vi "night time stamp.vi"(8 "error in (no error)":errorcluster) -> (0 "error out":errorcluster, 2 "date time rec":T1)   [LabVIEW 2018]
uses:
  <vilib>/Utility/miscctls.llb/LVDateTimeRec.ctl
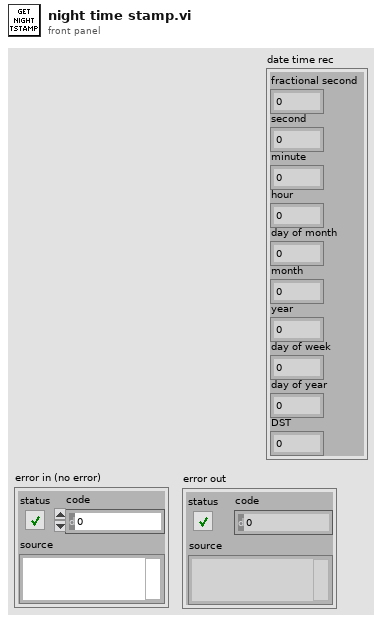
[diagram p1: front panel]
types:
  T1 = typedef "LVDateTimeRec.ctl" = cluster{"fractional second":dbl, "second":i32, "minute":i32, "hour":i32, "day of month":i32, "month":i32, "year":i32, "day of week":i32, "day of year":i32, "DST":i32}
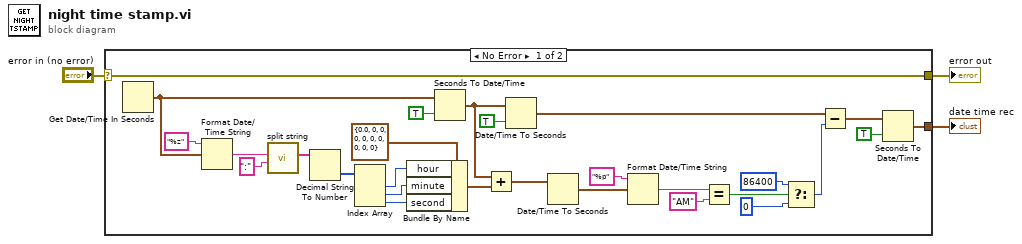
[diagram p0: block diagram]
diagram:
  n1 = case shown="No Error" "error in (no error)" {
    selector: "error in (no error)" -> [w31 w32]
    tunnel: [w31 w32] -> w2
    tunnel: [w6 _] -> w1
    frame No Error {
      n2 = Get Date/Time In Seconds() -> (seconds since 1Jan1904=w21:timestamp)
      n3 = Format Date/Time String(time format string (%c)="%z", seconds (now)=w21) -> (date/time string=w28:string)  [unwired: 1 in]
      n4 = call "split string.vi"("search string"=":", "String"=w28) -> ("strings array"=w26:string[])  [unwired: 8 in, 1 out]
      n5 = Decimal String To Number(string=w26) -> (number=w25:i32[])  [unwired: 2 in, 1 out]
      n6 = Index Array(array=w25) -> (element #1=w24:i32, element #2=w23:i32, element #3=w22:i32)  [unwired: 3 in]
      n7 = Bundle By Name(cluster=T1 {"fractional second"=0.0, "second"=0, "minute"=0, "hour"=0, "day of month"=0, "month"=0, "year"=0, "day of week"=0, "day of year"=0, "DST"=0} ("date time rec 2"), "hour"=w24, "minute"=w23, "second"=w22) -> (w19:T1)
      n8 = Seconds To Date/Time(time stamp (now)=w21, to UTC (F)=TRUE) -> (date time rec=w11:T1)
      n9 = Add(x=w11, y=w19) -> (x+y=w12:T1)
      n10 = Date/Time To Seconds(1:TRUE ("is UTC (F)"), 2:w11) -> (0:w8:timestamp)
      n11 = Date/Time To Seconds(2:w12) -> (0:w18:timestamp)  [unwired: 1 in]
      n12 = Format Date/Time String(time format string (%c)="%p", seconds (now)=w18) -> (date/time string=w13:string)  [unwired: 1 in]
      n13 = Equal?(x=w13, y="AM") -> (x = y?=w15:bool)
      n14 = Select(t=86400, s=w15, f=0) -> (s? t:f=w16:i32)
      n15 = Subtract(x=w8, y=w16) -> (x-y=w7:timestamp)
      n16 = Seconds To Date/Time(time stamp (now)=w7, to UTC (F)=TRUE) -> (date time rec=w6:T1)
    }
    frame Error {
    }
  }
  "error out" <- w2
  "date time rec" <- w1
